vi "SET Enqueuers Array 2 Dispatch Message.vi"(8 "error in (no error)":errorcluster, 10 "Enqueuers Array":refnum<class "Message Enqueuer.lvclass">[](array[class]), 11 "Child_2_Class in":refnum<class "Child_2_Class.lvclass">=refnum) -> (0 "error out":errorcluster, 3 "Child_2_Class out":refnum<class "Child_2_Class.lvclass">)   [LabVIEW 2023, in "Actor_Child_2.lvlib" / "Child_2_Class.lvclass"]
uses:
  Child_2_Class.lvclass
  <vilib>/ActorFramework/Message Enqueuer/Message Enqueuer.lvclass
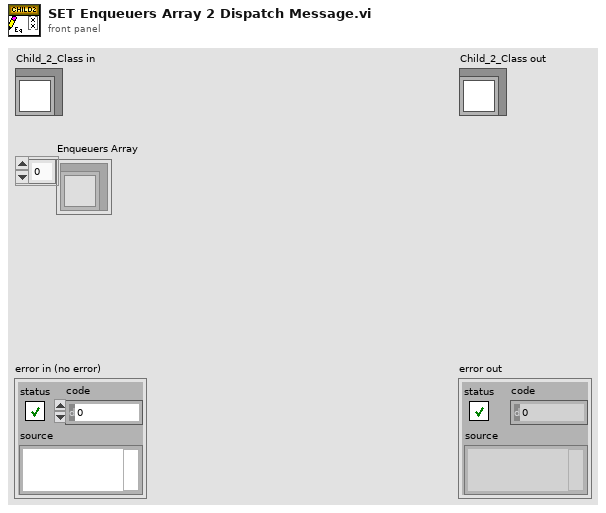
[diagram p1: front panel]
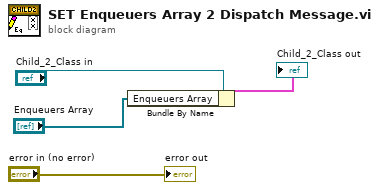
[diagram p0: block diagram]
diagram:
  n1 = Bundle By Name(cluster="Child_2_Class in", "Enqueuers Array"="Enqueuers Array") -> (→"Child_2_Class out":cluster{})
  "error out" <- "error in (no error)"
